vi "ListControlUI.vi"() -> ()   [LabVIEW 2015, in "List_UI.lvclass"]
uses:
  List_UI.lvclass
  <vilib>/Utility/error.llb/Error Cluster From Error Code.vi
  <vilib>/ErrorRing/Error Ring.xnode
  resources/_excel/Excel.lvclass
panel:
  in  "Next":bool
  in  "Last":bool
  in  "Stop":bool
  in  "Table Control":string[][](table)
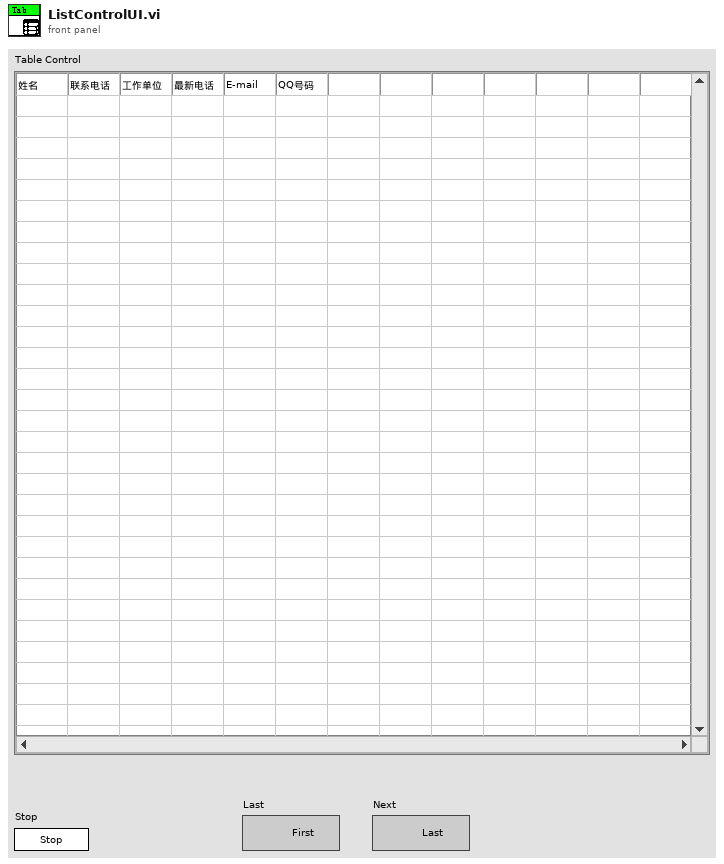
[diagram p1: front panel]
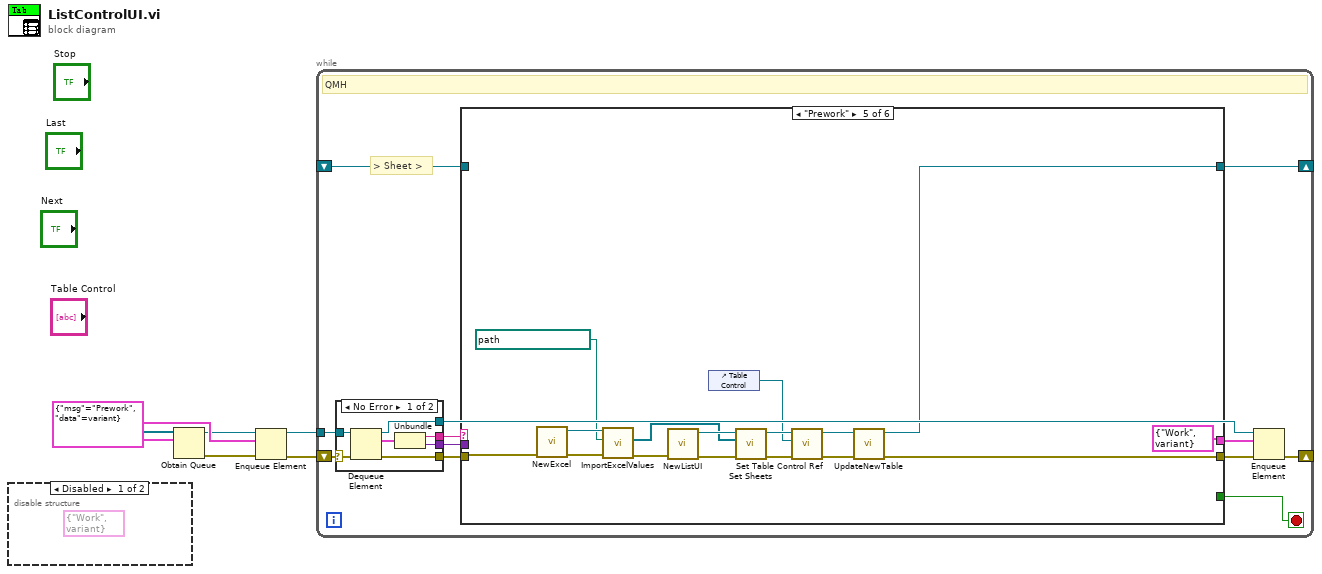
[diagram p0: block diagram]
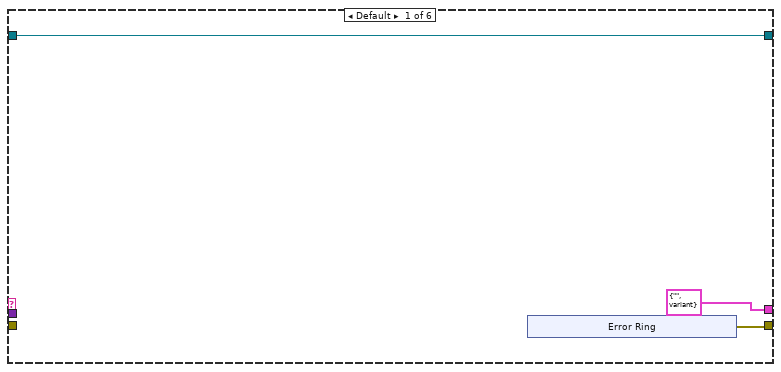
[diagram p3: hidden frame]
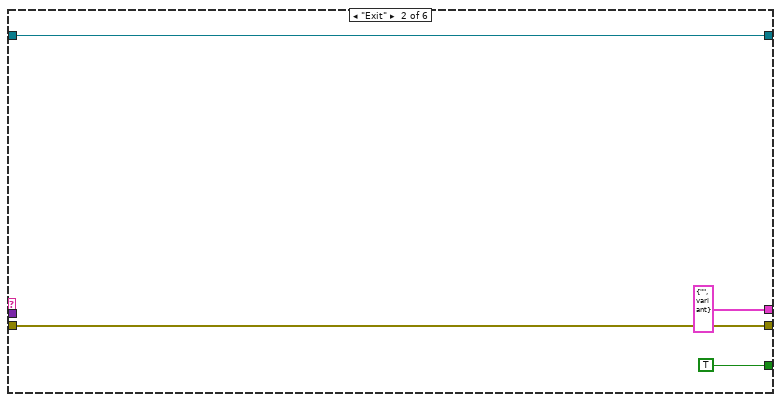
[diagram p4: hidden frame]
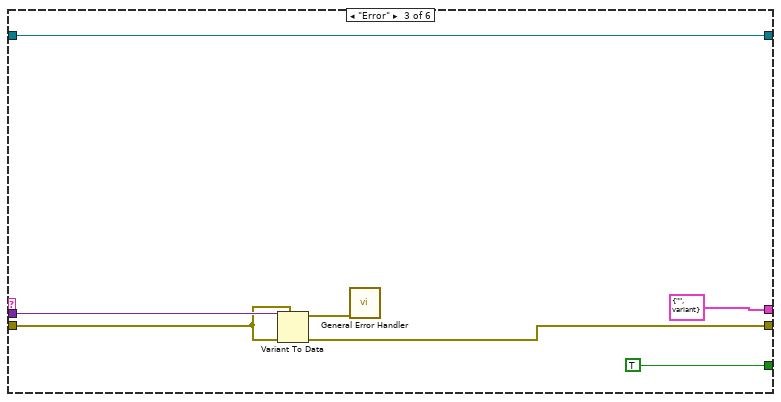
[diagram p5: hidden frame]
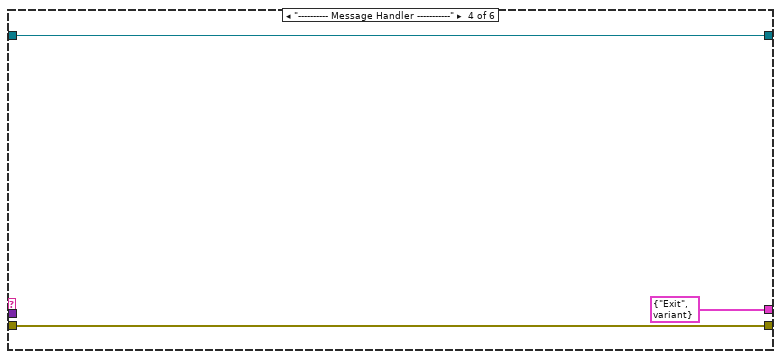
[diagram p6: hidden frame]
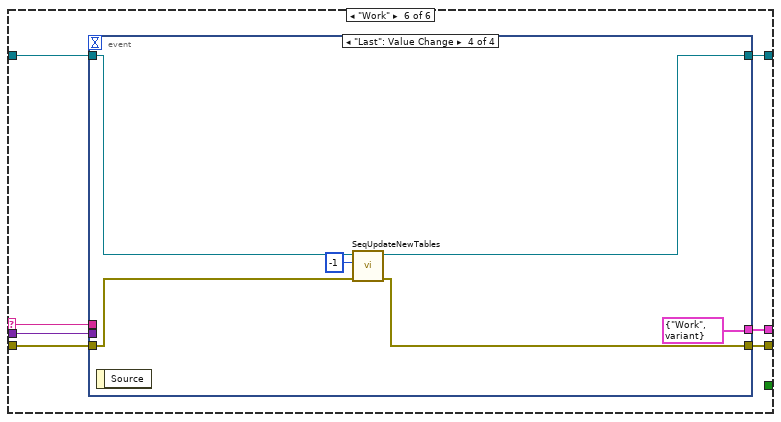
[diagram p7: hidden frame]
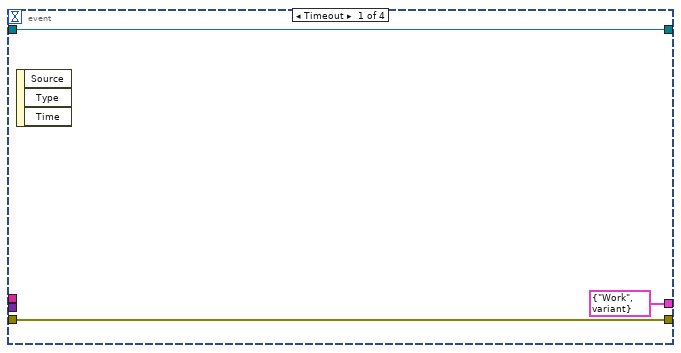
[diagram p8: hidden frame]
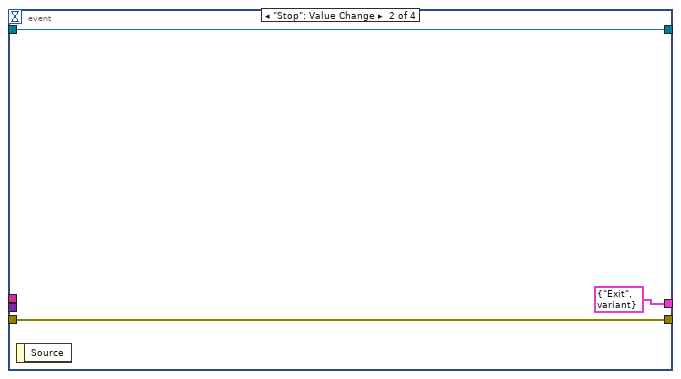
[diagram p9: hidden frame]
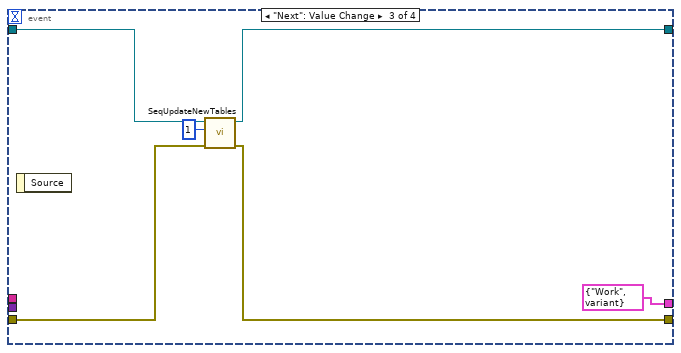
[diagram p10: hidden frame]
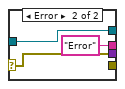
[diagram p11: hidden frame]
diagram:
  w3 = cluster{"msg":string, "data":variant} {"msg"="Prework", "data"=variant}
  n1 = disable-structure shown="Disabled" {
    frame Disabled {
      (unwired) cluster{"msg":string, "data":variant} {"msg"="Work", "data"=variant}
    }
    frame Enabled {
    }
  }
  n2 = Obtain Queue(element data type=w3) -> (queue out=w1:refnum<queue>, error out=w2:errorcluster)  [unwired: 4 in, 1 out]
  n3 = Enqueue Element(queue=w1, element=w3, error in (no error)=w2) -> (queue out=w4:refnum<queue>, error out=w5:errorcluster)  [unwired: 1 in, 1 out]
  n4 = while {
    tunnel: w4 -> [w16]
    shift-right: [w11] -> _
    shift-left: w5 -> [w17]
    shift-right: [w7] -> _
    shift-left: _ -> [w6]
    stop <- w8 stop-if-true
    # "> Sheet >"
    # "QMH"
    n5 = case shown="No Error" w17 {
      selector: w17 -> [w86 w90]
      tunnel: w16 -> [w87 w88]
      tunnel: [w85 _] -> w15
      tunnel: [w83 "Error" ("msg")] -> w14
      tunnel: [w82 w90] -> w13
      tunnel: [w81 w88] -> w10
      frame No Error {
        n6 = Dequeue Element(queue=w87, error in (no error)=w86) -> (queue out=w81:refnum<queue>, element=w84:cluster{"msg":string, "data":variant}, error out=w85:errorcluster)  [unwired: 1 in, 1 out]
        n7 = Unbundle(w84) -> ("msg"=w83:string, "data"=w82:variant)
      }
      frame Error {
      }
    }
    n8 = case shown="\"Prework\"" w14 {
      selector: w14 -> [_ _ _ _ _ w60]
      tunnel: w15 -> [_ w29 w35 w39 w54 w62]
      tunnel: w13 -> [_ _ w36 _ _ w61]
      tunnel: [w20 w29 w33 w39 w40 w59] -> w12
      tunnel: [cluster{"msg":string, "data":variant} {"msg"="", "data"=variant} cluster{"msg":string, "data":variant} {"msg"="", "data"=variant} cluster{"msg":string, "data":variant} {"msg"="", "data"=variant} cluster{"msg":string, "data":variant} {"msg"="Exit", "data"=variant} cluster{"msg":string, "data":variant} {"msg"="Work", "data"=variant} w58] -> w9
      tunnel: [_ TRUE TRUE _ _ _] -> w8
      tunnel: [w18 w26 w30 w37 w41 w56] -> w7
      tunnel: w6 -> [w18 w26 w30 w37 _ w57]
      frame Default {
        n9 = xnode "Error Ring"() -> ("error out"=w20:errorcluster)
      }
      frame "Exit" {
      }
      frame "Error" {
        n10 = Variant To Data(error in=w35, type=w35, Variant=w36) -> (data=w34:errorcluster, error out=w33:errorcluster)
        n11 = call <vilib>:"General Error Handler.vi"("error in (no error)"=w34) -> ()  [unwired: 10 in, 5 out]
      }
      frame "---------- Message Handler -----------" {
      }
      frame "Prework" {
        n12 = call "NewExcel.vi"("error in (no error)"=w54) -> ("error out"=w52:errorcluster, "Excel out"=w53:refnum<class "Excel.lvclass">)  [unwired: 9 in]
        n13 = call "ImportExcelValues.vi"("error in (no error)"=w52, "ExcelPath"=path "E:/LabVIEW相关/LabVIEW项目/机电学院档案管理系统_201603/LV/Archive/resources/_excel/学籍档案模板.xlsx" ("Path"), "Excel in"=w53) -> ("error out"=w50:errorcluster, "Sheets"=w47:refnum<class "List.lvclass">[])  [unwired: 6 in, 1 out]
        n14 = call "NewListUI.vi"("error in (no error)"=w50) -> ("error out"=w48:errorcluster, "List_UI out"=w49:refnum<class "List_UI.lvclass">)  [unwired: 9 in]
        n15 = control-ref of="Table Control"() -> (w44:refnum<vi>)
        n16 = call "Set Sheets.vi"("error in (no error)"=w48, "Sheets"=w47, "List_UI in"=w49) -> ("error out"=w45:errorcluster, "List_UI out"=w46:refnum<class "List_UI.lvclass">)  [unwired: 7 in]
        n17 = call "Set Table Control Ref.vi"("error in (no error)"=w45, "Table Control"=w44, "List_UI in"=w46) -> ("error out"=w42:errorcluster, "List_UI out"=w43:refnum<class "List_UI.lvclass">)  [unwired: 7 in]
        n18 = call "UpdateNewTable.vi"("error in (no error)"=w42, "List_UI in"=w43) -> ("error out"=w40:errorcluster, "List_UI out"=w41:refnum<class "List_UI.lvclass">)  [unwired: 8 in]
      }
      frame "Work" {
        n19 = event shown="[3] \"Last\": Value Change" {
          selector: _ -> [_ _ _ _]
          dyn-events: _ -> [_ _ _ _]
          timeout: _ -> [_ _ _ _]
          tunnel: w62 -> [w65 w68 w72 w79]
          tunnel: w61 -> [_ _ _ _]
          tunnel: w60 -> [_ _ _ _]
          tunnel: [w65 w68 w70 w76] -> w59
          tunnel: [cluster{"msg":string, "data":variant} {"msg"="Work", "data"=variant} cluster{"msg":string, "data":variant} {"msg"="Exit", "data"=variant} cluster{"msg":string, "data":variant} {"msg"="Work", "data"=variant} cluster{"msg":string, "data":variant} {"msg"="Work", "data"=variant}] -> w58
          tunnel: w57 -> [w63 w66 w74 w80]
          tunnel: [w63 w66 w71 w77] -> w56
          event Timeout {
            n20 = event-data() -> ()  [unwired: 1 in, 3 out]
          }
          event "Stop": Value Change {
            n21 = event-data() -> ()  [unwired: 1 in, 1 out]
          }
          event "Next": Value Change {
            n22 = event-data() -> ()  [unwired: 1 in, 1 out]
            n23 = call "SeqUpdateNewTables.vi"("error in (no error)"=w72, "Delta"=1, "List_UI in"=w74) -> ("error out"=w70:errorcluster, "List_UI out"=w71:refnum<class "List_UI.lvclass">)  [unwired: 7 in]
          }
          event "Last": Value Change {
            n24 = event-data() -> ()  [unwired: 1 in, 1 out]
            n25 = call "SeqUpdateNewTables.vi"("error in (no error)"=w79, "Delta"=-1, "List_UI in"=w80) -> ("error out"=w76:errorcluster, "List_UI out"=w77:refnum<class "List_UI.lvclass">)  [unwired: 7 in]
          }
        }
      }
    }
    n26 = Enqueue Element(queue=w10, element=w9, error in (no error)=w12) -> (error out=w11:errorcluster)  [unwired: 1 in, 2 out]
  }
